vi "dll_cuda_v2_80.vi"(6 "n_stream":i32, 7 "rdp_mean":sgl[][](array[numeric]), 8 "yc":sgl[][](array[numeric]), 9 "xc":sgl[][](array[numeric]), 10 "rdp_profile":sgl[][][](array[numeric]), 11 "img_mat 4d":sgl[][][][](array[numeric])) -> (0 "yc out":sgl[][](array[numeric]), 1 "xc out":sgl[][](array[numeric]), 2 "rdp_profile out":sgl[][][](array[numeric]), 3 "rdp_mean out":sgl[][](array[numeric]))   [LabVIEW 2017]
uses:
  Users/user/Documents/Visual Studio 2015/Projects/cuda_QI_v3/x64/Release/cuda_QI_v2.dll
panel:
  out "n_stream 2":i32
  out "n_frame":i32
  out "arraySize":i32
  out "img_mat":sgl[][][][](array[numeric])
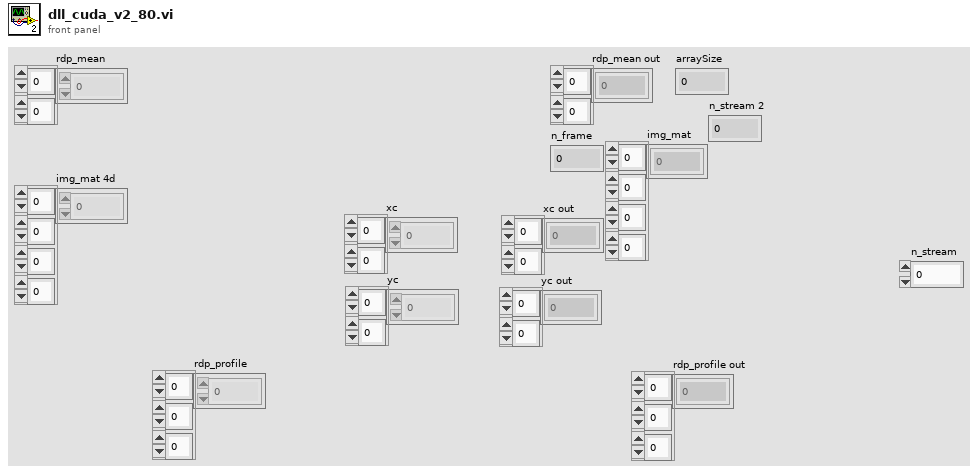
[diagram p1: front panel]
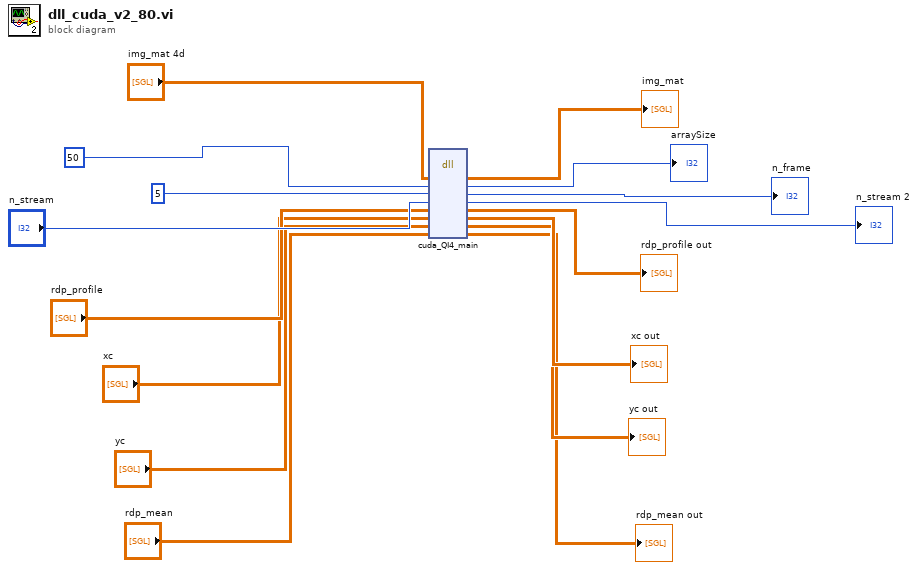
[diagram p0: block diagram]
diagram:
  n1 = dll-call lib="C:/Users/user/Documents/Visual Studio 2015/Projects/cuda_QI_v3/x64/Release/cuda_QI_v2.dll" fn="cuda_QI4_main"("img_mat"="img_mat 4d", "arraySize"=50, "n_frame"=5, "n_stream"="n_stream", "rdp_profile"="rdp_profile", "xc"="xc", "yc"="yc", "rdp_mean"="rdp_mean") -> ("img_mat"=→"img_mat":sgl[][][][], "arraySize"=→"arraySize":i32, "n_frame"=→"n_frame":i32, "n_stream"=→"n_stream 2":i32, "rdp_profile"=→"rdp_profile out":sgl[][][], "xc"=→"xc out":sgl[][], "yc"=→"yc out":sgl[][], "rdp_mean"=→"rdp_mean out":sgl[][])  [unwired: 4 in, 2 out]
